vi "Add_File_NumExt.vi"(9 "Extension":string, 10 "file or folder exists?":bool, 11 "Path In":path) -> (3 "Path Out":path)   [LabVIEW 2012]
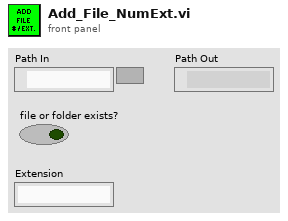
[diagram p1: front panel]
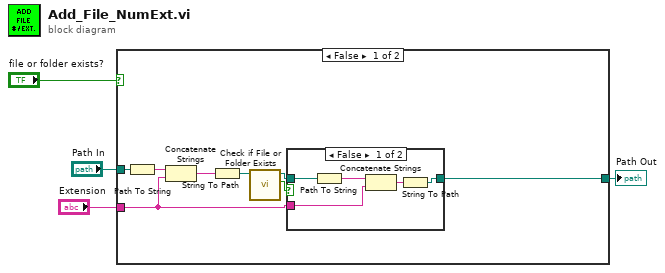
[diagram p0: block diagram]
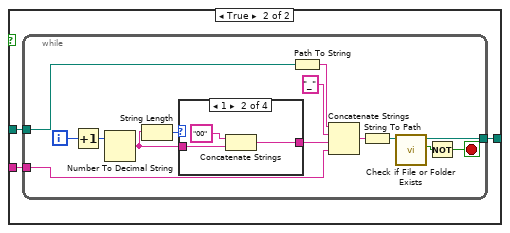
[diagram p3: hidden frame]
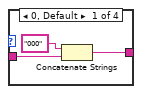
[diagram p4: hidden frame]
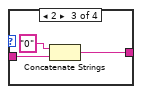
[diagram p5: hidden frame]
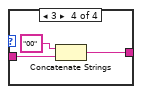
[diagram p6: hidden frame]
diagram:
  n1 = case shown="False" "file or folder exists?" {
    tunnel: "Path In" -> [w8 w21]
    tunnel: [w12 w19] -> w3
    tunnel: "Extension" -> [w5 w20]
    frame False {
      n2 = Path To String(path=w8) -> (string=w11:string)
      n3 = Concatenate Strings(w11, w5) -> (w9:string)
      n4 = String To Path(string=w9) -> (path=w10:path)
      n5 = call <vilib>:"Check if File or Folder Exists.vi"("path"=w10) -> ("file or folder exists?"=w7:bool, "dup path"=w6:path)  [unwired: 8 in, 1 out]
      n6 = case shown="False" w7 {
        tunnel: [w15 w18] -> w12
        tunnel: w6 -> [w14 w18]
        tunnel: w5 -> [w13 _]
        frame False {
          n7 = Path To String(path=w14) -> (string=w17:string)
          n8 = Concatenate Strings(w17, w13) -> (w16:string)
          n9 = String To Path(string=w16) -> (path=w15:path)
        }
        frame True {
        }
      }
    }
    frame True {
      n10 = while {
        tunnel: w21 -> [w28]
        tunnel: [w27] -> w19
        tunnel: w20 -> [w26]
        i -> [w29]
        stop <- w30 stop-if-true
        n11 = Increment(x=w29) -> (x+1=w25:i32)
        n12 = Number To Decimal String(number=w25) -> (decimal integer string=w23:string)  [unwired: 1 in]
        n13 = String Length(string=w23) -> (length=w24:i32)
        n14 = case shown="1" w24 {
          tunnel: w23 -> [w37 w41 w43 w45]
          tunnel: [w36 w40 w42 w47] -> w22
          frame 0, Default {
            n15 = Concatenate Strings("000", w37) -> (w36:string)
          }
          frame 1 {
            n16 = Concatenate Strings("00" ("string"), w41) -> (w40:string)
          }
          frame 2 {
            n17 = Concatenate Strings("0" ("string"), w43) -> (w42:string)
          }
          frame 3 {
            n18 = Concatenate Strings("00" ("string"), w45) -> (w47:string)
          }
        }
        n19 = Path To String(path=w28) -> (string=w35:string)
        n20 = Concatenate Strings(w35, "_", w22, w26) -> (w33:string)
        n21 = String To Path(string=w33) -> (path=w32:path)
        n22 = call <vilib>:"Check if File or Folder Exists.vi"("path"=w32) -> ("file or folder exists?"=w31:bool, "dup path"=w27:path)  [unwired: 8 in, 1 out]
        n23 = Not(x=w31) -> (.not. x?=w30:bool)
      }
    }
  }
  "Path Out" <- w3
